vi "Chamber controller Dec 2 2016 new turbo.vi"() -> ()   [LabVIEW 2014]
uses:
  <vilib>/Instr/_visa.llb/VISA Configure Serial Port (Instr).vi
  Environmental Chamber LabVIEW and Instruments/Drivers and Software/Keithley 2100 Series/Public/Configure/Configure 2 Wire Resistance.vi
  <vilib>/Utility/file.llb/Write To Spreadsheet File (string).vi
  <vilib>/Utility/file.llb/Read From Spreadsheet File (string).vi
  Environmental Chamber LabVIEW and Instruments/Drivers and Software/keithley_6430/Keithley 6430/Public/Data/Read (Single Point).vi
  Environmental Chamber LabVIEW and Instruments/Drivers and Software/LabVIEW 8.2 Drivers/keithley_24xx/Keithley 24XX/Public/Data/Read (Single Point).vi
  Environmental Chamber LabVIEW and Instruments/Drivers and Software/keithley_24xx/Keithley 24XX/Keithley 24XX.lvlib
  Environmental Chamber LabVIEW and Instruments/Drivers and Software/keithley_6430/Keithley 6430/Keithley 6430.lvlib
  Environmental Chamber LabVIEW and Instruments/Drivers and Software/Keithley 2100 Series/Keithley 2100 Series.lvlib
panel:
  in  "Arduino COMs":T1={"Arduino 1"="COM23", "Arduino 2"="COM24", "Arduino 3"="COM25", "Arduino 4"="COM26", "Arduino 5"="COM27", "Arduino 6"="COM28"}
  out "saving data?":bool
  out "ArduinoQCM\ncluster":T2 caption="Arduino QCM" {"6" format="%_8g"; "5" format="%_8g"; "4" format="%_8g"; "3" format="%_8g"; "2" format="%_8g"; "1" format="%#_10g"}
  in  "Data logging settings":T3={"Save during sequence only"=TRUE, "Save now"=FALSE, "sec between data points"=0.0, "Current data file path"=path "", "Save sample names"={"QCM1"="", "QCM2"="", "QCM3"="", "QCM4"="", "QCM5"="", "QCM6"="", "SRS"="", "K-2420"="", "K-6430"="", "K-2100"=""}, "Experiment Notes"=""} {"sec between data points" min=0.0 max=30.0 format="%#_13g"}
  in  "Sequence cluster":T4={"Save sequence"=FALSE, "Clear sequence"=FALSE, "Import sequence file"=FALSE, "Tare elapsed time"=TRUE, "Run Sequence"=FALSE, "Stop program when sequence ends"=TRUE, "User-defined\nsequence"=[], "Sequence end time"="", "Sequence\npreview"=[], "Current\nstep"=0} caption="Sequence settings"
  in  "Pressure parameters cluster":T5={"valve % open"=100.0, "Desired pressure"=0.0, "Vapor sccm"=0.0, "Gas sccm"=0.0, "Valve mode"=enum."% Open", "Pressure Mode"=enum."Abs. pressure", "analyte partial pressure"=23.8, "Turbo pump\nauto on"=TRUE, "Valve position (%)"=0.0, "read pressure"=0.0, "read vapor flow"=0.0, "read gas flow"=0.0, "pressure chart"={"pressure"=0.0}} caption="Pressure settings" {"read gas flow" format="%#_3g"; "read vapor flow" format="%#_3g"; "read pressure" format="%#_7f"; "Valve position (%)" format="%#_3g"; "analyte partial pressure" min=0.0 max=100.0 step=5.0; "Gas sccm" min=0 max=200 step=5; "Vapor sccm" min=0 max=200 step=5; "Desired pressure" min=0.0 max=760.0 step=5.0; "valve % open" min=0.0 max=100.0 step=5.0 format="%#_2f"}
  out "J-KEM temp chart":dbl(graph)
  out "Elapsed time (min)":dbl
  out "State date/time":string caption="Start time"
  out "K-2100 (Ohm)":cluster{"Measurement":dbl}(graph) caption="K-2100"
  out "K-6430":cluster{"Measurement":dbl}(graph)
  out "K-2420":cluster{"Resistance":sgl}(graph)
  in  "Gate time (sec)":enum16{"0.1", "1.0 ", "10"}(ring)=enum."1.0 "
  out "Hz":dbl format="%#.7f"
  out "QCM plot":T6(graph)
  in  "Stop":bool
  in  "Clear all charts":bool
  out "O2 sensor output":dbl[](array[numeric]) caption="atm\nTorr"
  in  "rapidox O2 Sensor":bool
  in  "setnag O2 Pump":bool
  in  "Baud Rate 2":i32(ring)=2 items=["2400", "4800", "9600", "19200", "38400", "57600", "115200"]
  in  "Com Port":i32(ring) items=["Com 1", "Com 2", "Com 3", "Com 4", "Com 5", "Com 6", "COM 7", "COM 8", "COM 9", "COM 10", "COM 11", "COM 12", "com 13", "COM 14"]
  in  "Com Port 2":i32(ring) items=["Com 1", "Com 2", "Com 3", "Com 4", "Com 5", "Com 6", "COM 7", "COM 8", "COM 9", "COM 10", "COM 11", "COM 12", "com 13", "COM 14"]
  out "Waveform Chart":cluster{dbl}(graph)
  out "O2 Concentration (PPM)":dbl
  out "Waveform Chart 6":cluster{dbl}(graph)
  # "SRS"
  # "Currently Unused"
  # "100%"
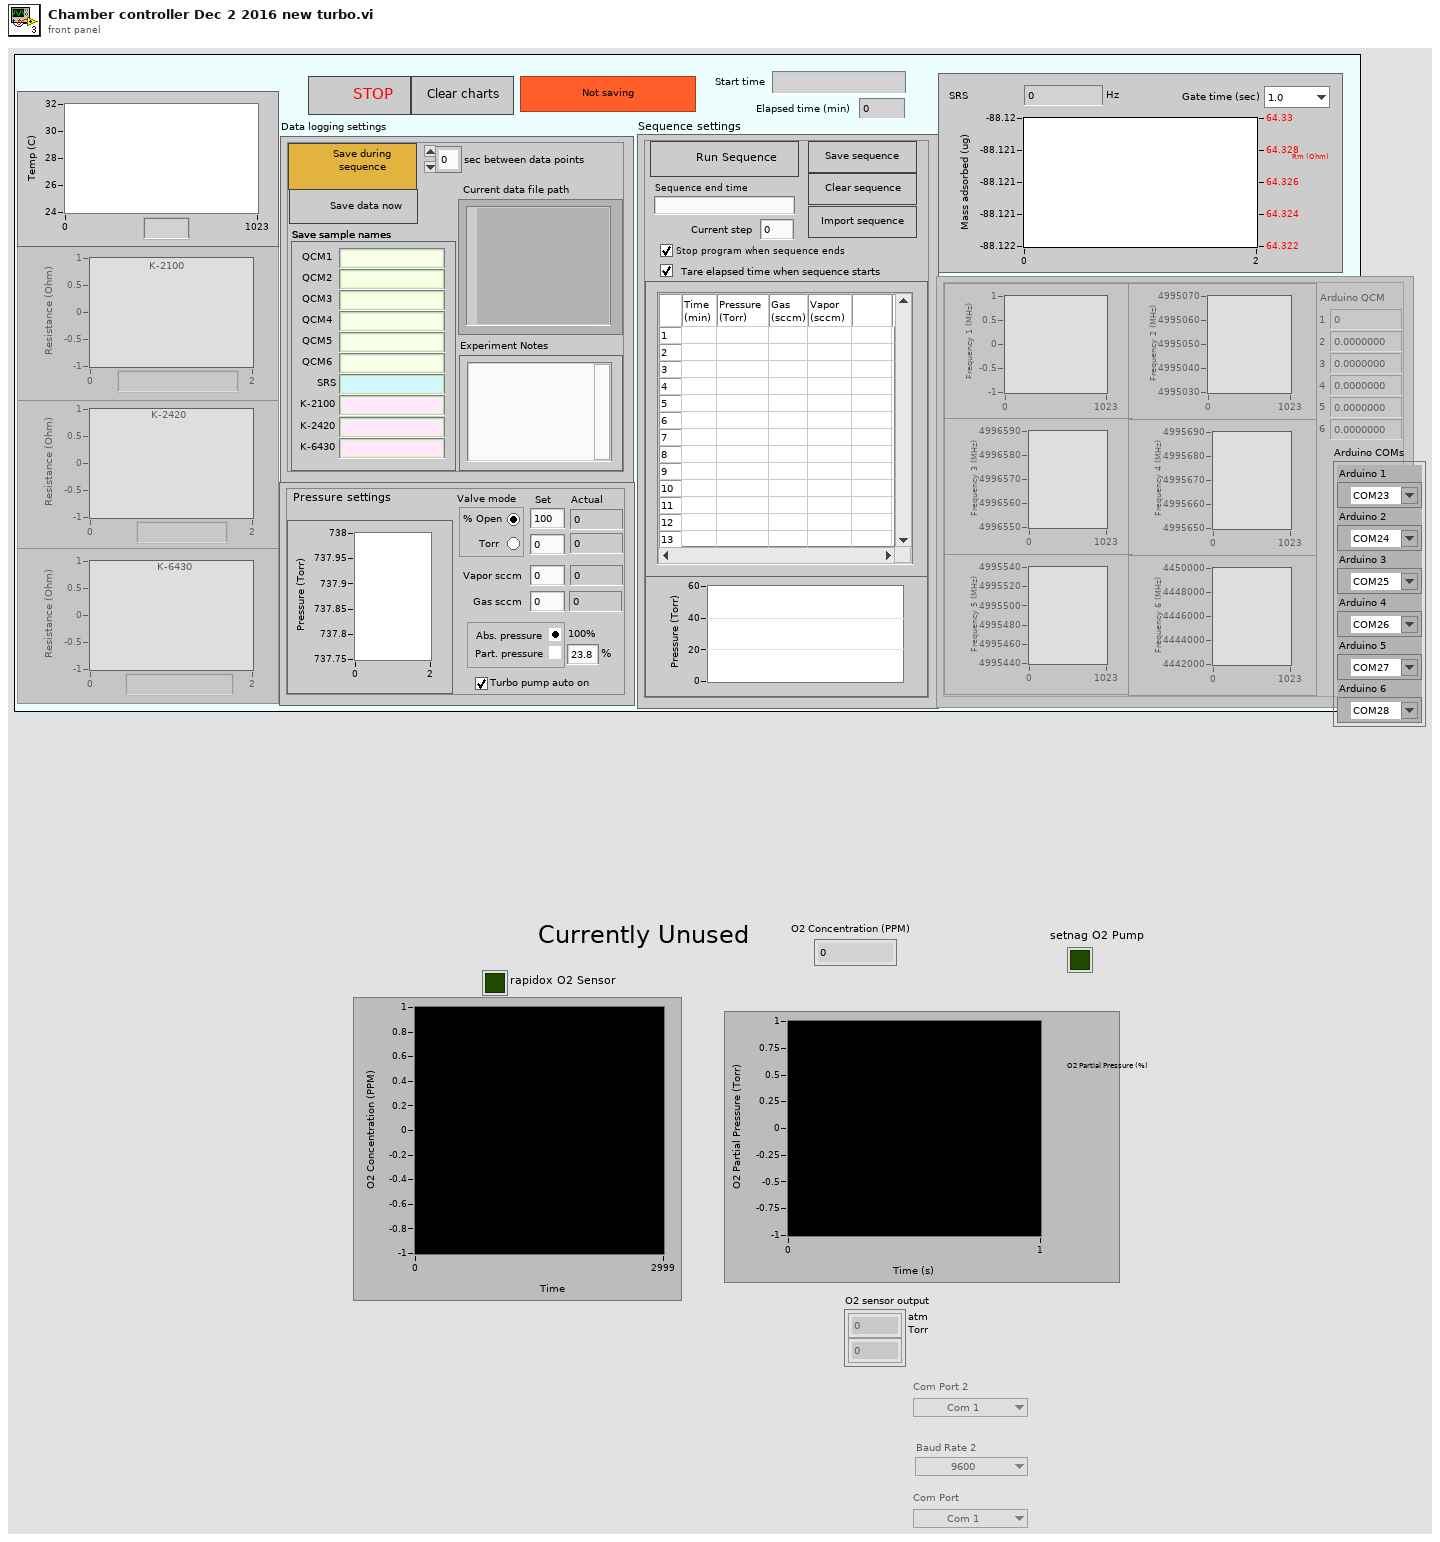
[diagram p1: front panel]
types:
  T1 = cluster{"Arduino 1":refnum<visa-resource-name>, "Arduino 2":refnum<visa-resource-name>, "Arduino 3":refnum<visa-resource-name>, "Arduino 4":refnum<visa-resource-name>, "Arduino 5":refnum<visa-resource-name>, "Arduino 6":refnum<visa-resource-name>}
  T2 = cluster{"arduino qcm 1":dbl, "1":dbl, "arduino qcm 2":dbl, "2":dbl, "arduino qcm 3":dbl, "3":dbl, "arduino qcm 4":dbl, "4":dbl, "arduino qcm 5":dbl, "5":dbl, "arduino qcm 6":dbl, "6":dbl}
  T3 = cluster{"Save during sequence only":bool, "Save now":bool, "sec between data points":dbl, "Current data file path":path, "Save sample names":cluster{"QCM1":string, "QCM2":string, "QCM3":string, "QCM4":string, "QCM5":string, "QCM6":string, "SRS":string, "K-2420":string, "K-6430":string, "K-2100":string}, "Experiment Notes":string}
  T4 = cluster{"Save sequence":bool, "Clear sequence":bool, "Import sequence file":bool, "Tare elapsed time":bool, "Run Sequence":bool, "Stop program when sequence ends":bool, "User-defined\nsequence":string[][], "Sequence end time":string, "Sequence\npreview":cluster{dbl[], dbl[]}[], "Current\nstep":i32}
  T5 = cluster{"valve % open":dbl, "Desired pressure":dbl, "Vapor sccm":sgl, "Gas sccm":sgl, "Valve mode":enum32{"% Open", "Torr "}, "Pressure Mode":enum32{"Abs. pressure", " Part. pressure"}, "analyte partial pressure":dbl, "Turbo pump\nauto on":bool, "Valve position (%)":dbl, "read pressure":dbl, "read vapor flow":dbl, "read gas flow":dbl, "pressure chart":cluster{"pressure":dbl}}
  T6 = cluster{"Numeric Control":dbl, "Resistance out":dbl}
  T7 = cluster{"Keithley 6430":bool, "J-KEM":bool, "Keithley 2420":bool, "Keithley 2100":bool, "SRS QCM":bool, "Pressure control":bool, "Arduino":bool}
  T8 = enum8{"Enabled", "Disabled", "Disabled and Grayed Out"}
  T9 = enum16{"open", "open or create", "create or replace", "create", "open (read only)"}
  T10 = enum16{"no parity", "odd parity", "even parity", "mark parity", "space parity"}
  T11 = cluster{"String":string, "String":string, "String":string}
  T12 = cluster{bool, "task out":refnum<k21>, "error out":errorcluster, "task out":refnum<k21>, "error out":errorcluster, "turbo pump":refnum<visa-resource-name>, "error out":errorcluster}
  T13 = cluster{bool, "task out":refnum<k21>, "error out":errorcluster, "task out":refnum<k21>, "error out":errorcluster, "VISA resource name out":refnum<visa-resource-name>, "error out":errorcluster}
  T14 = cluster{bool, "VISA resource name":refnum<visa-resource-name>, "error out":errorcluster}
  T15 = cluster{bool, "VISA resource name out":refnum<visa-resource-name>, "error out":errorcluster}
  T16 = cluster{"VISA resource name out":refnum<visa-resource-name>, "error out":errorcluster, "VISA resource name out":refnum<visa-resource-name>, "error out":errorcluster, "VISA resource name out":refnum<visa-resource-name>, "error out":errorcluster, "VISA resource name out":refnum<visa-resource-name>, "error out":errorcluster, "VISA resource name out":refnum<visa-resource-name>, "error out":errorcluster, "VISA resource name out 2":refnum<visa-resource-name>, "error out 2":errorcluster}
  T17 = cluster{"Boolean":bool, "VISA resource name out":refnum<visa-resource-name>, "error out":errorcluster}
  T18 = cluster{bool, "VISA out":refnum<visa-resource-name>, "error out":errorcluster}
  T19 = cluster{"Boolean":bool, "VISA out":refnum<visa-resource-name>, "error out":errorcluster}
  T20 = cluster{"Numeric Control":dbl, "Cluster":cluster{"Numeric Control":dbl}, "String":string, "error out":errorcluster}
  T21 = cluster{bool, "Com Port":i32, "Numeric Control out":dbl}
  T22 = cluster{"Arduino address":refnum<visa-resource-name>, "error in (no error)":errorcluster, "Arduino address 2":refnum<visa-resource-name>, "error in (no error) 2":errorcluster, "Arduino address 3":refnum<visa-resource-name>, "error in (no error) 3":errorcluster, "Arduino address 4":refnum<visa-resource-name>, "error in (no error) 4":errorcluster, "Arduino address 5":refnum<visa-resource-name>, "error in (no error) 5":errorcluster, "Arduino address 6":refnum<visa-resource-name>, "error in (no error) 6":errorcluster}
  T23 = cluster{"mean":string, "mean":string, "mean":string, "mean":string, "mean":string, "mean":string}
  T24 = cluster{"String data out":string, string, string, string}
  T25 = cluster{"valve % open":dbl, "Desired pressure":dbl, "Vapor sccm":sgl, "Gas sccm":sgl, "Valve mode":enum32{"% Open", "Torr "}, "Pressure Mode":enum32{"Abs. pressure", " Part. pressure"}, "analyte partial pressure":dbl}
  T26 = cluster{"User-defined\nsequence":string[][], "Present (s)":dbl, "current  step # in":i32, "sequence end time in":timestamp}
  T27 = cluster{"current  step # in":i32, "sequence end time in":timestamp, "Boolean":bool}
  T28 = cluster{"press/RH/gas/vapor":cluster{"pressure":string, "RH":string, "gas flow":string, "vapor flow":string}, "Cluster":cluster{"Valve position (%)":dbl, "read pressure":dbl, "read vapor flow":dbl, "read gas flow":dbl}}
  T29 = cluster{"Boolean":bool, "task out":refnum<k21>, "error out":errorcluster, "task out":refnum<k21>, "error out":errorcluster, "VISA resource name out":refnum<visa-resource-name>, "error out":errorcluster}
  T30 = cluster{"f":dbl, "f":dbl, "f":dbl, "f":dbl, "f":dbl}[]
  T31 = cluster{"pressure":string, "RH":string, "gas flow":string, "vapor flow":string}
  T32 = cluster{"Valve position (%)":dbl, "read pressure":dbl, "read vapor flow":dbl, "read gas flow":dbl}
  T33 = cluster{"mean":dbl, "mean":dbl, "mean":dbl, "mean":dbl, "mean":dbl, "mean":dbl}
  T34 = cluster{"QCM1":string, "QCM2":string, "QCM3":string, "QCM4":string, "QCM5":string, "QCM6":string, "SRS":string, "K-2420":string, "K-6430":string, "K-2100":string}
  T35 = cluster{"mean":dbl, "mean":dbl, "mean":dbl, "mean":dbl, "mean":dbl, "mean":dbl, "mean":dbl, "mean":dbl, "mean":dbl, "mean":dbl, "mean":dbl, "mean":dbl}
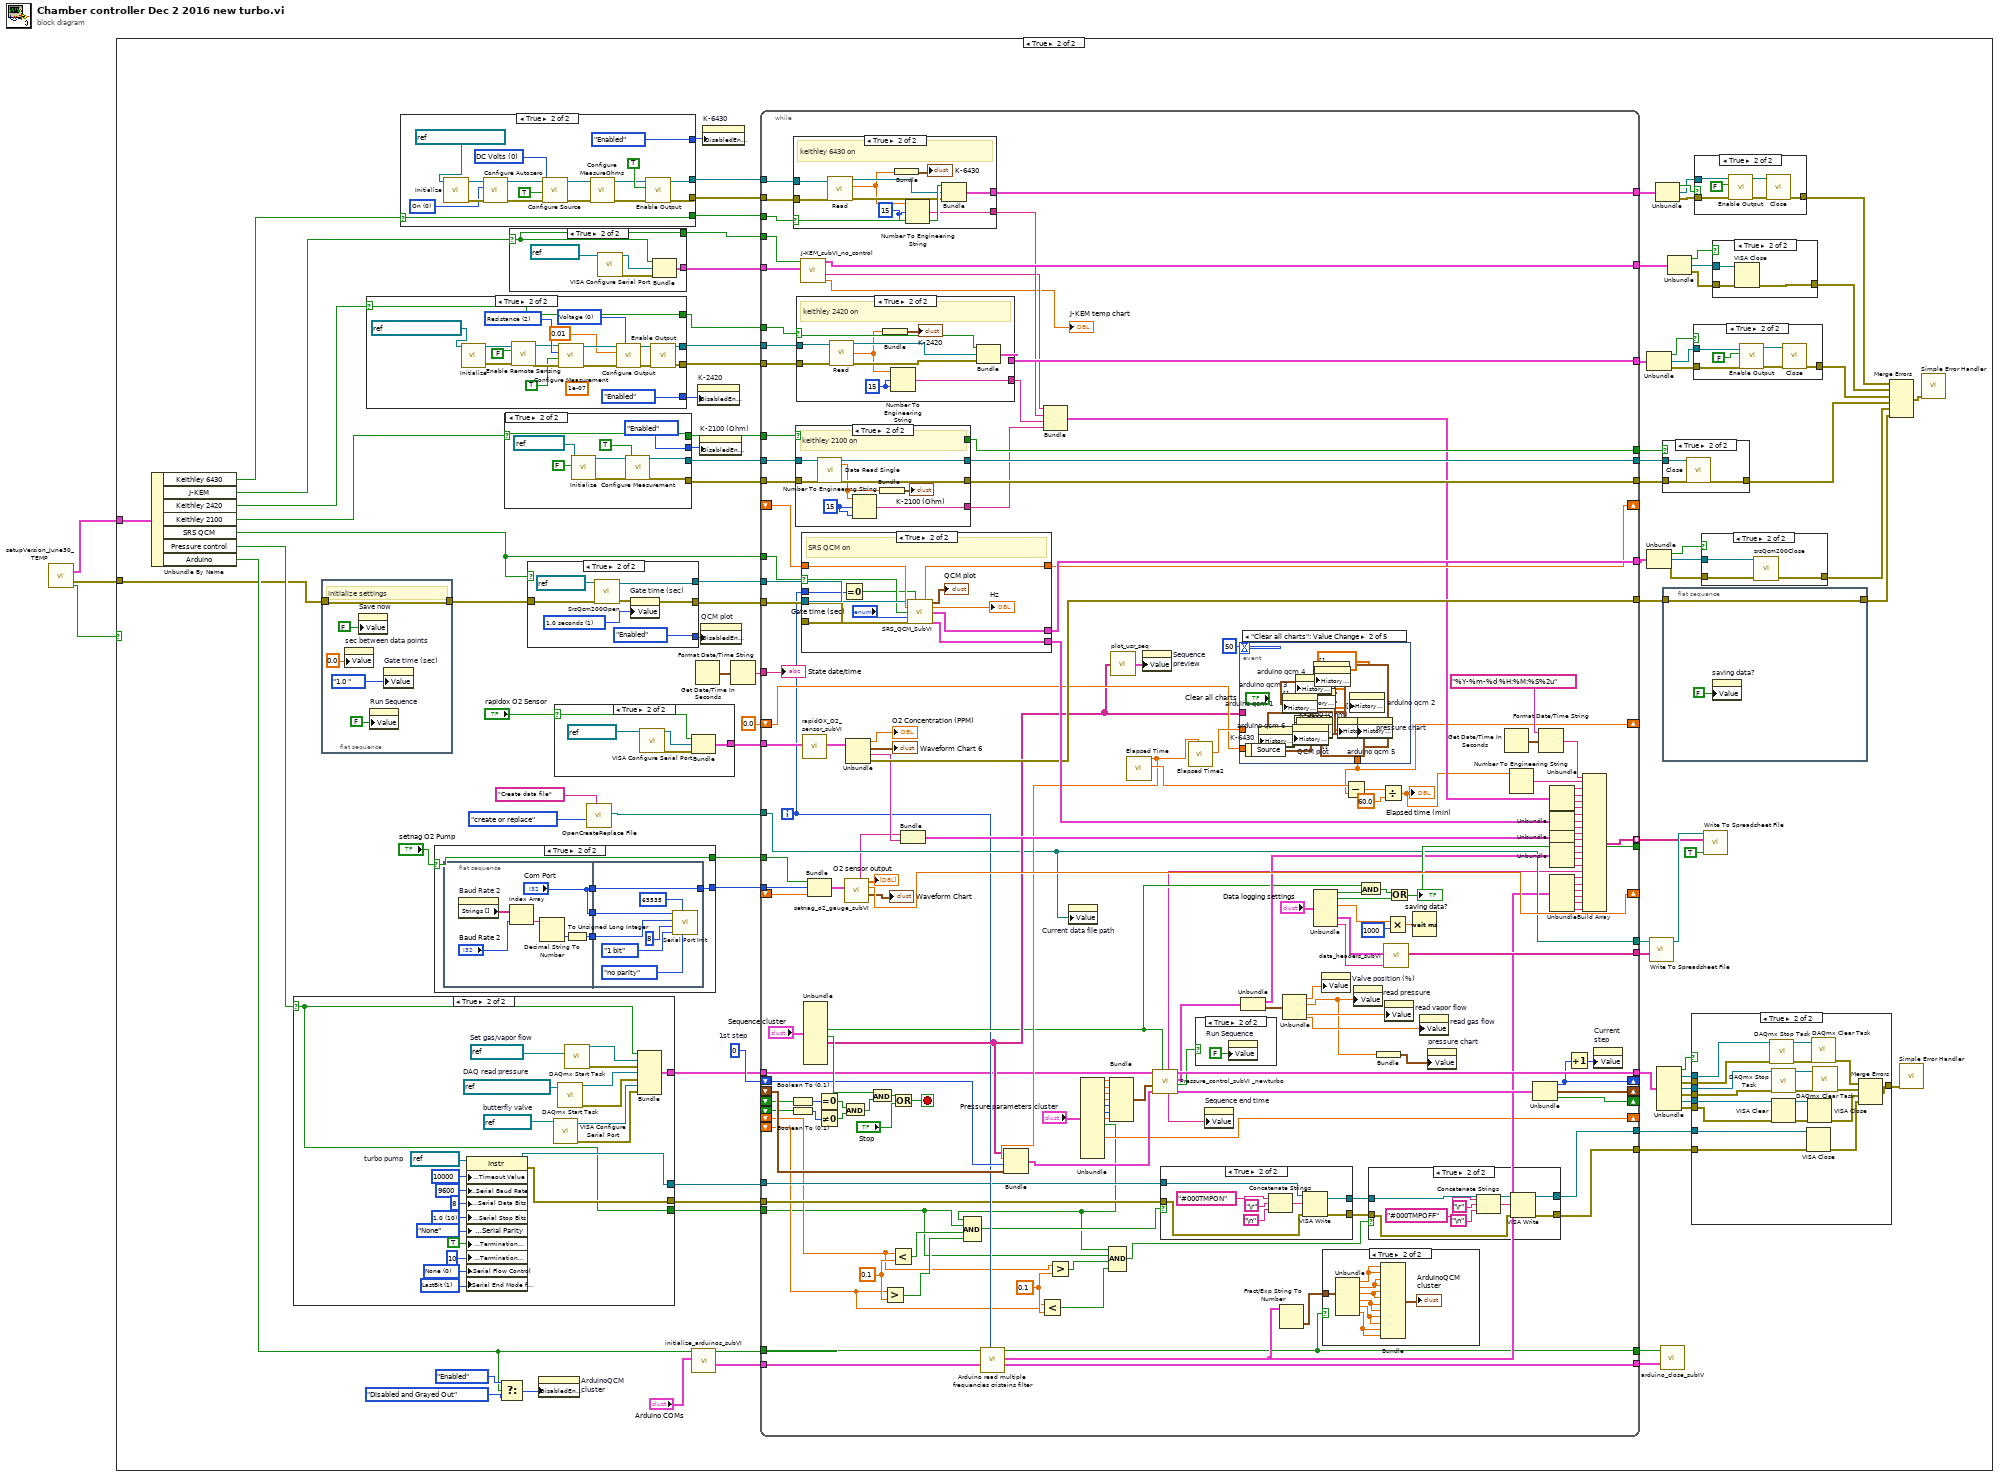
[diagram p0: block diagram]
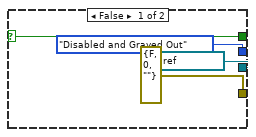
[diagram p4: hidden frame]
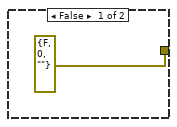
[diagram p5: hidden frame]
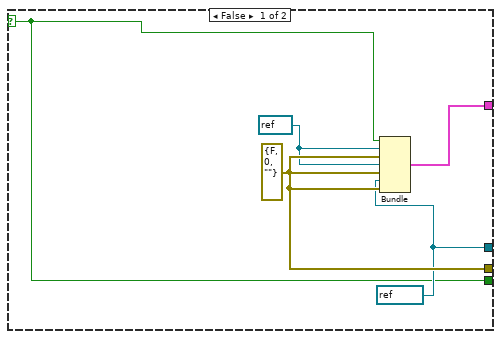
[diagram p6: hidden frame]
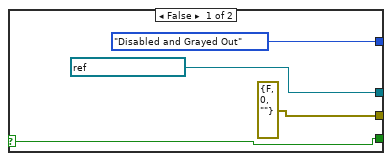
[diagram p8: hidden frame]
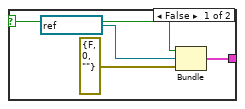
[diagram p9: hidden frame]
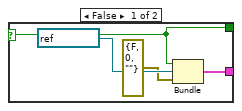
[diagram p11: hidden frame]
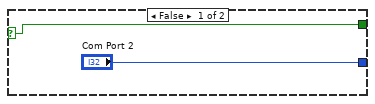
[diagram p12: hidden frame]
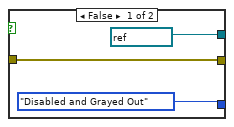
[diagram p14: hidden frame]
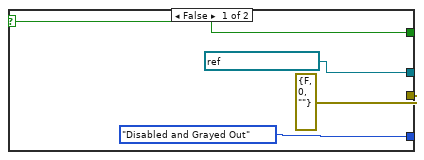
[diagram p16: hidden frame]
diagram:
  n1 = call "setupVersion_June30_TEMP.vi"() -> ("Instruments on/off"=w1:T7, "error IO"=w2:errorcluster, "OK"=w3:bool)  [unwired: 13 in]
  n2 = case shown="True" w3 {
    tunnel: w2 -> [_ w17]
    tunnel: w1 -> [_ w27]
    frame False {
    }
    frame True {
      w34 = 0  # 1st step
      n3 = Unbundle By Name(w27) -> ("Keithley 6430"=w26:bool, "J-KEM"=w25:bool, "Keithley 2420"=w24:bool, "Keithley 2100"=w23:bool, "SRS QCM"=w22:bool, "Pressure control"=w21:bool, "Arduino"=w20:bool)
      n4 = case shown="True" w21 {
        selector: w21 -> [w142 w147]
        tunnel: [w146 w148] -> w15
        tunnel: [w145 w150] -> w7
        tunnel: [w143 w149] -> w8
        tunnel: [w142 w147] -> w6
        frame False {
          w143 = refnum<visa-resource-name> refnum ("turbo pump")
          w144 = refnum<k21> refnum ("task out")
          w145 = errorcluster {"status"=FALSE, "code"=0, "source"=""} ("error out")
          n5 = Bundle(w142, "task out"=w144, "error out"=w145, "task out"=w144, "error out"=w145, "turbo pump"=w143, "error out"=w145) -> (w146:T12)  [unwired: 1 in]
        }
        frame True {
          w154 = u16 1 items=["None", "LastBit", "TermChar"] ("Serial Settings:Serial End Mode for Reads")
          w152 = u16 0 items=["None", "XON/XOFF", "RTS/CTS", "XON/XOFF & RTS/CTS", "DTR/DSR", "XON/XOFF & DTR/DSR"] ("flow control (0:none)")
          w155 = u16 10 items=["1.0"=10, "1.5"=15, "2.0"=20] ("stop bits (10: 1 bit)")
          w151 = refnum<visa-resource-name> "COM7"  # turbo pump
          w167 = refnum<visa-resource-name> "COM5"  # butterfly valve
          w168 = refnum<k21> "Setflow"  # Set gas/vapor flow
          w169 = refnum<k21> "AllDaqReadings"  # DAQ read pressure
          n6 = property class="Instr"(reference=w151, "General Settings:Timeout Value"=u32 10000 ("timeout (10sec)"), "Serial Settings:Serial Baud Rate"=u32 9600 ("baud rate (9600)"), "Serial Settings:Serial Data Bits"=u16 8 ("data bits (8)"), "Serial Settings:Serial Stop Bits"=w155, "Serial Settings:Serial Parity"=enum16{"None", "Odd", "Even", "Mark", "Space"}."None" ("parity (0:none)"), "Message Based Settings:Termination Character Enable"=TRUE ("Enable Termination\nChar (T)"), "Message Based Settings:Termination Character"=u8 10 ("termination char\n(0xA = '\\n' = LF)"), "Serial Settings:Serial Flow Control"=w152, "Serial Settings:Serial End Mode for Reads"=w154) -> (reference out=w149:refnum<visa-resource-name>, error out=w150:errorcluster)  [unwired: 1 in]
          n7 = call-poly "VISA Configure Serial Port"("VISA resource name"=w167) -> ("VISA resource name out"=w162:refnum<visa-resource-name>, "error out"=w161:errorcluster)  [unwired: 13 in]
          n8 = call <vilib>:"DAQmx Start Task.vi"("task/channels in"=w169) -> ("task out"=w164:refnum<k21>, "error out"=w163:errorcluster)  [unwired: 13 in]
          n9 = call <vilib>:"DAQmx Start Task.vi"("task/channels in"=w168) -> ("task out"=w166:refnum<k21>, "error out"=w165:errorcluster)  [unwired: 13 in]
          n10 = Bundle(w147, "task out"=w166, "error out"=w165, "task out"=w164, "error out"=w163, "VISA resource name out"=w162, "error out"=w161) -> (w148:T13)  [unwired: 1 in]
        }
      }
      n11 = flat-sequence {
        tunnel: [w98] -> w16
        tunnel: w17 -> [w98]
        frame #0 {
          # "initialize settings"
          n12 = property on="sec between data points" class="DigNum (strict)"("Value"=0.0) -> ()  [unwired: 2 in, 2 out]
          n13 = property on="Save now" class="Bool (strict)"("Value"=FALSE) -> ()  [unwired: 2 in, 2 out]
          n14 = property on="Run Sequence" class="Bool (strict)"("Value"=FALSE) -> ()  [unwired: 2 in, 2 out]
          n15 = property on="Gate time (sec)" class="Enum (strict)"("Value"=enum16{"0.1", "1.0 ", "10"}."1.0 " ("Gate time (sec)")) -> ()  [unwired: 2 in, 2 out]
        }
      }
      n16 = case shown="True" w24 {
        selector: w24 -> [w261 w265]
        tunnel: [refnum<visa-resource-name> "GPIB1::24::INSTR" ("VISA resource name") w274] -> w95
        tunnel: [errorcluster {"status"=FALSE, "code"=0, "source"=""} ("error out") w269] -> w94
        tunnel: [T8."Disabled and Grayed Out" ("Disabled") T8."Enabled" ("Disabled")] -> w58
        tunnel: [w261 w265] -> w51
        frame False {
        }
        frame True {
          (unwired) 1e-07 ("Manual Range (1.0)")
          w276 = u16 0 items=["Voltage", "Current"] ("Source Mode  (0: Voltage)")
          w281 = u16 2 items=["Volts", "Current", "Resistance"] ("Function (0: Volts)")
          n17 = call "Initialize.vi"("VISA resource name"=refnum<visa-resource-name> "GPIB1::24::INSTR") -> ("error out"=w270:errorcluster, "VISA resource name out"=w273:refnum<visa-resource-name>)  [unwired: 9 in]
          n18 = call "Enable Remote Sensing.vi"("error in (no error)"=w270, "Enable Remote Sensing (T: Enable)"=FALSE ("4-wire?"), "VISA resource name"=w273) -> ("error out"=w271:errorcluster, "VISA resource name out"=w272:refnum<visa-resource-name>)  [unwired: 7 in]
          n19 = call "Configure Measurement.vi"("error in (no error)"=w271, "Enable Auto Range (T:Enable)"=TRUE, "Function (0: Volts)"=w281, "VISA resource name"=w272) -> ("error out"=w280:errorcluster, "VISA resource name out"=w279:refnum<visa-resource-name>)  [unwired: 6 in]
          n20 = call "Configure Output.vi"("Source Mode  (0: Voltage)"=w276, "error in (no error)"=w280, "Output Level (0)"=0.01 ("Applied Voltage (V)"), "VISA resource name"=w279) -> ("error out"=w278:errorcluster, "VISA resource name out"=w277:refnum<visa-resource-name>)  [unwired: 6 in]
          n21 = call "Enable Output.vi"("error in (no error)"=w278, "VISA resource name"=w277) -> ("error out"=w269:errorcluster, "VISA resource name out"=w274:refnum<visa-resource-name>)  [unwired: 8 in]
        }
      }
      n22 = case shown="True" w26 {
        selector: w26 -> [w177 w181]
        tunnel: [refnum<visa-resource-name> "GPIB0::29::INSTR" ("VISA resource name") w192] -> w64
        tunnel: [errorcluster {"status"=FALSE, "code"=0, "source"=""} ("error out") w193] -> w63
        tunnel: [T8."Disabled and Grayed Out" ("Disabled") T8."Enabled" ("Disabled")] -> w57
        tunnel: [w177 w181] -> w50
        frame False {
        }
        frame True {
          w182 = u16 0 items=["DC Volts", "DC Current"] ("Source Function (0: DC Volts)")
          w189 = u16 0 items=["On", "Off", "Once"] ("Autozero  (0: On)")
          n23 = call "Initialize.vi"("VISA resource name"=refnum<visa-resource-name> "GPIB0::29::INSTR") -> ("error out"=w190:errorcluster, "VISA resource name out"=w191:refnum<visa-resource-name>)  [unwired: 4 in, 5 out]
          n24 = call "Configure Autozero.vi"("error in (no error)"=w190, "Autozero  (0: On)"=w189, "VISA resource name"=w191) -> ("error out"=w185:errorcluster, "VISA resource name out"=w187:refnum<visa-resource-name>)  [unwired: 7 in]
          n25 = call "Configure Source.vi"("error in (no error)"=w185, "Auto Range (T:Enable)"=TRUE, "Source Function (0: DC Volts)"=w182, "VISA resource name"=w187) -> ("error out"=w184:errorcluster, "VISA resource name out"=w186:refnum<visa-resource-name>)  [unwired: 6 in]
          n26 = call "Configure MeasureOhms.vi"("error in (no error)"=w184, "VISA resource name"=w186) -> ("error out"=w197:errorcluster, "VISA resource name out"=w195:refnum<visa-resource-name>)  [unwired: 4 in, 4 out]
          n27 = call "Enable Output.vi"("error in (no error)"=w197, "Enable Output (F:Off)"=TRUE ("Output (F:Off)"), "VISA resource name"=w195) -> ("error out"=w193:errorcluster, "VISA resource name out"=w192:refnum<visa-resource-name>)  [unwired: 7 out]
        }
      }
      n28 = case shown="True" "setnag O2 Pump" {
        selector: "setnag O2 Pump" -> [w220 w222]
        tunnel: ["Com Port 2" w223] -> w91
        tunnel: [w220 w222] -> w39
        frame False {
        }
        frame True {
          n29 = flat-sequence {
            tunnel: ["Com Port"] -> w226
            tunnel: [w228] -> w225
            tunnel: ["Com Port"] -> w224
            tunnel: w226 -> [w234]
            tunnel: w225 -> [w233]
            tunnel: w224 -> [w235]
            tunnel: [w235] -> w223
            frame #0 {
              n30 = property on="Baud Rate 2" class="Ring (strict)"() -> ("Strings []"=w230:string[])  [unwired: 2 in, 2 out]
              n31 = Index Array(array=w230, index="Baud Rate 2") -> (element=w231:string)
              n32 = Decimal String To Number(string=w231) -> (number=w229:i32)  [unwired: 2 in, 1 out]
              n33 = To Unsigned Long Integer(number=w229) -> (unsigned 32bit integer=w228:u32)
            }
            frame #1 {
              n34 = call <vilib>:"Serial Port Init.vi"("parity"=T10."no parity", "buffer size"=u16 65535, "stop bits"=enum16{"1 bit", "1.5 bits", "2 bits"}."1 bit", "data bits"=u16 8, "baud rate"=w233, "port number"=w234) -> ()  [unwired: 1 in, 1 out]
            }
          }
        }
      }
      n35 = Select(t=T8."Enabled" ("Disabled"), s=w20, f=T8."Disabled and Grayed Out" ("Disabled")) -> (s? t:f=w31:T8)
      n36 = case shown="True" w23 {
        selector: w23 -> [w110 w115]
        tunnel: [refnum<visa-resource-name> "K-2100" ("VISA resource name out") w118] -> w48
        tunnel: [errorcluster {"status"=FALSE, "code"=0, "source"=""} ("error out") w117] -> w47
        tunnel: [w110 w115] -> w46
        tunnel: [T8."Disabled and Grayed Out" ("Disabled") T8."Enabled" ("Disabled")] -> w41
        frame False {
        }
        frame True {
          n37 = call "Initialize.vi"("VISA resource name"=refnum<visa-resource-name> "K-2100", "Reset? (T: Reset)"=FALSE) -> ("VISA resource name out"=w119:refnum<visa-resource-name>, "error out"=w116:errorcluster)  [unwired: 16 in]
          n38 = call-poly "Configure Measurement.vi"("VISA resource name"=w119, "error in (no error)"=w116, "Auto Range? (T: Auto)"=TRUE) -> ("VISA resource name out"=w118:refnum<visa-resource-name>, "error out"=w117:errorcluster)  [unwired: 15 in]
        }
      }
      n39 = case shown="True" w25 {
        selector: w25 -> [w211 w216]
        tunnel: [w212 w217] -> w80
        tunnel: [w211 w216] -> w74
        frame False {
          n40 = Bundle(w211, "VISA resource name"=refnum<visa-resource-name> "COM3", "error out"=errorcluster {"status"=FALSE, "code"=0, "source"=""}) -> (w212:T14)  [unwired: 1 in]
        }
        frame True {
          n41 = call-poly "VISA Configure Serial Port"("VISA resource name"=refnum<visa-resource-name> "COM3") -> ("VISA resource name out"=w218:refnum<visa-resource-name>, "error out"=w215:errorcluster)  [unwired: 13 in]
          n42 = Bundle(w216, "VISA resource name out"=w218, "error out"=w215) -> (w217:T15)  [unwired: 1 in]
        }
      }
      n43 = case shown="True" w22 {
        tunnel: [refnum<visa-resource-name> "COM6" ("VISA in") w250] -> w93
        tunnel: [w245 w247] -> w92
        tunnel: w16 -> [w245 w252]
        tunnel: [T8."Disabled and Grayed Out" ("Disabled") T8."Enabled" ("Disabled")] -> w59
        frame False {
        }
        frame True {
          w249 = u16 1 items=["0.1 seconds", "1.0 seconds", "10.0 seconds"] ("Gate time")
          n44 = call "SrsQcm200Open.vi"("error in"=w252, "VISA in"=refnum<visa-resource-name> "COM6") -> ("error out"=w248:errorcluster, "VISA out"=w250:refnum<visa-resource-name>)  [unwired: 3 in]
          n45 = property on="Gate time (sec)" class="Enum (strict)"(error in=w248, "Value"=w249) -> (error out=w247:errorcluster)  [unwired: 1 in, 1 out]
        }
      }
      n46 = property on="ArduinoQCM\ncluster" class="Clust (strict)"("DisabledEnum"=w31) -> ()  [unwired: 2 in, 2 out]
      n47 = case shown="True" "rapidox O2 Sensor" {
        selector: "rapidox O2 Sensor" -> [w198 w203]
        tunnel: [w199 w204] -> w70
        frame False {
          n48 = Bundle(w198, "VISA resource name"=refnum<visa-resource-name> "COM7", "error out"=errorcluster {"status"=FALSE, "code"=0, "source"=""}) -> (w199:T14)  [unwired: 1 in]
        }
        frame True {
          n49 = call-poly "VISA Configure Serial Port"("VISA resource name"=refnum<visa-resource-name> "COM7") -> ("VISA resource name out"=w205:refnum<visa-resource-name>, "error out"=w202:errorcluster)  [unwired: 13 in]
          n50 = Bundle(w203, "VISA resource name out"=w205, "error out"=w202) -> (w204:T15)  [unwired: 1 in]
        }
      }
      n51 = call "OpenCreateReplace File.vi"("prompt"="Create data file", "function (open:0)"=T9."create or replace") -> ("new file path"=w49:path)  [unwired: 6 in, 3 out]
      n52 = call "initialize_arduinos_subVI.vi"("arduino 1-6 addresses"="Arduino COMs", "arduinos on?"=w20) -> ("arduino addresses/errors"=w35:T16, "arduinos on/off"=w55:bool)  [unwired: 8 in]
      n53 = Get Date/Time In Seconds() -> (seconds since 1Jan1904=w97:timestamp)
      n54 = property on="K-2420" class="WFChart (strict)"("DisabledEnum"=w58) -> ()  [unwired: 2 in, 2 out]
      n55 = property on="K-2100 (Ohm)" class="WFChart (strict)"("DisabledEnum"=w41) -> ()  [unwired: 2 in, 2 out]
      n56 = property on="QCM plot" class="WFChart (strict)"("DisabledEnum"=w59) -> ()  [unwired: 2 in, 2 out]
      n57 = property on="K-6430" class="WFChart (strict)"("DisabledEnum"=w57) -> ()  [unwired: 2 in, 2 out]
      n58 = Format Date/Time String(seconds (now)=w97) -> (date/time string=w38:string)  [unwired: 2 in]
      n59 = while {
        shift-right: [w443] -> _
        shift-left: _ -> [w374]
        tunnel: [w427] -> w56 mode=indexing if=w396
        tunnel: w51 -> [w432]
        tunnel: w95 -> [w442]
        tunnel: w94 -> [w441]
        tunnel: w93 -> [w440]
        tunnel: w92 -> [w439]
        tunnel: w22 -> [w438]
        tunnel: w39 -> [w376]
        tunnel: w91 -> [w377]
        tunnel: [w437] -> w88
        tunnel: [w436] -> w84
        tunnel: w80 -> [w435]
        tunnel: [w434] -> w79
        tunnel: w74 -> [w433]
        tunnel: w70 -> [w385]
        tunnel: [w381] -> w19
        tunnel: [w318] -> w69
        tunnel: w49 -> [w318]
        shift-right: [w425] -> _
        shift-left: _ -> [w426]
        tunnel: w64 -> [w431]
        tunnel: w63 -> [w430]
        tunnel: [w429] -> w62
        tunnel: [w396] -> _
        tunnel: w55 -> [w306]
        tunnel: w35 -> [w309]
        tunnel: [w305] -> w53
        tunnel: [w307] -> w54
        tunnel: [w413] -> w52
        tunnel: w50 -> [w408]
        tunnel: w48 -> [w395]
        tunnel: w47 -> [w394]
        tunnel: w46 -> [w393]
        tunnel: [w392] -> w45
        tunnel: [w391] -> w44
        tunnel: [w390] -> w43
        shift-right: [w368] -> _
        shift-left: 0.0 ("Elapsed Time (s)") -> [w369]
        tunnel: w38 -> [w359]
        tunnel: w15 -> [w302]
        shift-right: [w314] -> _
        shift-left: w34 -> [w332]
        shift-right: [w338] -> _
        shift-left: _ -> [w336]
        shift-right: [w337] -> _
        shift-left: _ -> [w335]
        shift-left: _ -> [w334]
        tunnel: [w330] -> w33
        tunnel: w8 -> [w297]
        tunnel: w7 -> [w296]
        tunnel: w6 -> [w286]
        tunnel: [w291] -> w5
        tunnel: [w292] -> w4
        shift-right: [w301] -> _
        shift-left: _ -> [w288]
        shift-left: _ -> [w287]
        i -> [w304]
        stop <- w398 stop-if-true
        w290 = 0.1 ("y")
        w300 = 0.1 ("y")
        n60 = Boolean To (0,1)(Boolean=w335) -> (0, 1=w406:i16)
        n61 = Boolean To (0,1)(Boolean=w334) -> (0, 1=w405:i16)
        n62 = case "Keithley 6430" shown="True" w408 {
          selector: w408 -> [w498 w509]
          tunnel: w431 -> [w497 w506]
          tunnel: w430 -> [w496 w505]
          tunnel: ["" w508] -> w380
          tunnel: [w495 w507] -> w429
          frame False {
            # "keithley 6430 off"
            n63 = Bundle(w498, "VISA resource name out"=w497, "error out"=w496) -> (w495:T15)  [unwired: 1 in]
          }
          frame True {
            w500 = i16 15 ("width (-)")
            # "keithley 6430 on"
            n64 = call-poly "Read.vi"("error in (no error)"=w505, "VISA resource name"=w506) -> ("error out"=w504:errorcluster, "Measurement"=w502:dbl, "VISA resource name out"=w503:refnum<visa-resource-name>)  [unwired: 1 in, 6 out]
            n65 = Bundle("Measurement"=w502) -> (→"K-6430":cluster{"Measurement":dbl})  [unwired: 1 in]
            n66 = Number To Engineering String(2:w500, 3:w500, 4:w502) -> (0:w508:string)  [unwired: 1 in]
            n67 = Bundle(w509, "VISA resource name out"=w503, "error out"=w504) -> (w507:T15)  [unwired: 1 in]
          }
        }
        n68 = case shown="True" w393 {
          selector: w393 -> [w474 w479]
          tunnel: [w475 w486] -> w391
          tunnel: [w476 w485] -> w390
          tunnel: w395 -> [w475 w484]
          tunnel: w394 -> [w476 w483]
          tunnel: ["" w481] -> w378
          tunnel: [w474 w479] -> w392
          frame False {
            # "keithley 2100 off"
          }
          frame True {
            w478 = i16 15 ("width (-)")
            # "keithley 2100 on"
            n69 = call "Data Read Single.vi"("VISA resource name"=w484, "error in (no error)"=w483) -> ("VISA resource name out"=w486:refnum<visa-resource-name>, "Measurement"=w482:dbl, "error out"=w485:errorcluster)  [unwired: 15 in]
            n70 = Number To Engineering String ("elapsed time (min)")(2:w478, 3:w478, 4:w482) -> (0:w481:string)  [unwired: 1 in]
            n71 = Bundle("Measurement"=w482) -> (→"K-2100 (Ohm)":cluster{"Measurement":dbl})  [unwired: 1 in]
          }
        }
        n72 = case "Keithley 2420" shown="True" w432 {
          selector: w432 -> [w513 w522]
          tunnel: w442 -> [w512 w517]
          tunnel: w441 -> [w511 w516]
          tunnel: [w510 w520] -> w437
          tunnel: ["" w519] -> w379
          frame False {
            # "keithley 2420 off"
            n73 = Bundle(w513, "VISA resource name out"=w512, "error out"=w511) -> (w510:T15)  [unwired: 1 in]
          }
          frame True {
            w515 = i16 15 ("width (-)")
            # "keithley 2420 on"
            n74 = call-poly "Read.vi"("VISA resource name"=w517, "error in (no error)"=w516) -> ("VISA resource name out"=w523:refnum<visa-resource-name>, "Resistance"=w518:sgl, "error out"=w521:errorcluster)  [unwired: 7 in, 4 out]
            n75 = Bundle("Resistance"=w518) -> (→"K-2420":cluster{"Resistance":sgl})  [unwired: 1 in]
            n76 = Number To Engineering String(2:w515, 3:w515, 4:w518) -> (0:w519:string)  [unwired: 1 in]
            n77 = Bundle(w522, "VISA resource name out"=w523, "error out"=w521) -> (w520:T15)  [unwired: 1 in]
          }
        }
        n78 = call "J-KEM_subVI_no_control.vi"("Address in"=w435, "J-KEM on?"=w433) -> ("Temp (C)"=→"J-KEM temp chart":dbl, "String data out"=w367:string, "Address out"=w434:T17)  [unwired: 6 in, 1 out]
        n79 = case "SRS QCM" shown="True" w438 {
          selector: w438 -> [w527 w536]
          tunnel: w440 -> [w530 w538]
          tunnel: w439 -> [w529 w539]
          tunnel: [w528 w542] -> w436
          tunnel: w426 -> [w525 w541]
          tunnel: [w525 w540] -> w425
          tunnel: [T11 {"String"="", "String"="", "String"=""} ("M,F,MR output cluster") w535] -> w418
          tunnel: w304 -> [_ w532]
          frame False {
            # "SRS QCM off"
            n80 = Bundle(w527, "VISA out"=w530, "error out"=w529) -> (w528:T18)  [unwired: 1 in]
          }
          frame True {
            # "SRS QCM on"
            n81 = Equal To 0?(x=w532) -> (x = 0?=w533:bool)
            n82 = call "SRS_QCM_SubVI.vi"("VISA Refnum in"=w538, "first iteration?"=w533, "Frequency out 3"=w541, "Boolean 2"=w536, "Gate time"="Gate time (sec)", "error in (no error)"=w539) -> ("Frequency out 2"=w540:dbl, "Cluster"=→"QCM plot":T6, "Frequency out"=→"Hz":dbl, "Cluster 2"=w542:T19, "M,F,MR output cluster"=w535:T11)  [unwired: 2 in, 3 out]
          }
        }
        n83 = call "rapidOX_O2_sensor_subVI.vi"("rapid ox info in"=w385) -> ("rapidox info out"=w384:T20)  [unwired: 10 in]
        n84 = Unbundle("Sequence cluster") -> ("Run Sequence"=w324:bool, "Stop program when sequence ends"=w333:bool, "User-defined\nsequence"=w328:string[][])  [unwired: 7 out]
        n85 = Bundle(w376, "Com Port"=w377, "Numeric Control out"=w374) -> (w375:T21)  [unwired: 1 in]
        n86 = Equal To 0?(x=w406) -> (x = 0?=w403:bool)
        n87 = Not Equal To 0?(x=w405) -> (x != 0?=w404:bool)
        n88 = And(x=w403, y=w404) -> (x .and. y?=w397:bool)
        n89 = call "setnag_o2_gauge_subVI.vi"("setnag info in"=w375) -> ("Cluster"=→"Waveform Chart":cluster{"Numeric Control":dbl}, "Numeric Control out"=w443:dbl, "Array"=→"O2 sensor output":dbl[], "String"=w315:string)  [unwired: 7 in]
        n90 = Unbundle(w384) -> ("Numeric Control"=→"O2 Concentration (PPM)":dbl, "Cluster"=→"Waveform Chart 6":cluster{"Numeric Control":dbl}, "String"=w358:string, "error out"=w381:errorcluster)
        n91 = And(x=w333, y=w397) -> (x .and. y?=w372:bool)
        n92 = Greater?(x=w287, y=w300) -> (0:w299:bool)
        n93 = Less?(x=w288, y=w300) -> (x < y?=w298:bool)
        n94 = Or(x=w372, y="Stop") -> (x .or. y?=w398:bool)
        n95 = Bundle("String"=w315, "String"=w358) -> (w357:cluster{"String":string, "String":string})  [unwired: 1 in]
        n96 = call "Arduino read multiple frequencies cristains filter.vi"("main loop iteration number"=w304, "arduino addresses in"=w309, "arduinos on?"=w306) -> ("arduino addresses out"=w307:T22, "arduino frequencies out"=w308:T23, "arduinos on"=w305:bool)  [unwired: 6 in]
        n97 = Less?(x=w287, y=w290) -> (x < y?=w284:bool)
        n98 = Bundle("String data out"=w367, w380, w379, w378) -> (w373:T24)  [unwired: 1 in]
        n99 = Greater?(x=w288, y=w290) -> (0:w285:bool)
        n100 = property on="Current data file path" class="Path"("Value"=w318) -> ()  [unwired: 2 in, 2 out]
        n101 = Unbundle("Pressure parameters cluster") -> ("valve % open"=w347:dbl, "Desired pressure"=w349:dbl, "Vapor sccm"=w350:sgl, "Gas sccm"=w351:sgl, "Valve mode"=w352:enum32{"% Open", "Torr "}, "Pressure Mode"=w353:enum32{"Abs. pressure", " Part. pressure"}, "analyte partial pressure"=w354:dbl, "Turbo pump\nauto on"=w289:bool, "read pressure"=w301:dbl)  [unwired: 4 out]
        n102 = Compound Arithmetic op=AND(w289, w286, w298, w299) -> (w295:bool)
        n103 = Compound Arithmetic op=AND(w289, w286, w285, w284) -> (w283:bool)
        n104 = Bundle("valve % open"=w347, "Desired pressure"=w349, "Vapor sccm"=w350, "Gas sccm"=w351, "Valve mode"=w352, "Pressure Mode"=w353, "analyte partial pressure"=w354) -> (w346:T25)  [unwired: 1 in]
        n105 = call "plot_usr_seq.vi"("User-defined sequence"=w328) -> ("Sequence Preview"=w320:cluster{dbl[], dbl[]}[])
        n106 = call "Elapsed Time"() -> ("Present (s)"=w340:dbl, "Elapsed Time (s)"=w387:dbl)  [unwired: 12 in, 6 out]
        n107 = Bundle("User-defined\nsequence"=w328, "Present (s)"=w340, "current  step # in"=w332, "sequence end time in"=w336) -> (w341:T26)  [unwired: 1 in]
        n108 = property on="Sequence\npreview" class="XYGraph (strict)"("Value"=w320) -> ()  [unwired: 2 in, 2 out]
        n109 = call "Pressure_control_subVI _newturbo.vi"("Run Sequence"=w324, "user sequence, present (s) in, current step in, seq time in"=w341, "pressure parameters in"=w346, "pressure control on?/daq IDs/errors"=w302) -> ("current step # out, shift register time out, seq button on?"=w339:T27, "sequence over? USE THIS TO REINITIALIZE RUN SEQUENCE BUTTON SO PROGRAM ENDS"=w329:bool, "save press/RH/gasflow/vaporflow - read valve position/pressure/vaporflow/gasflow"=w327:T28, "pressure control on?/daq IDs/errors out"=w330:T29, "sequence end date/time string"=w331:string, "pressure_setpoint"=w311:string)  [unwired: 2 in]
        n110 = case shown="True" w295 {
          tunnel: w297 -> [w456 w459]
          tunnel: w296 -> [w455 w460]
          tunnel: [w456 w458] -> w294
          tunnel: [w455 w457] -> w293
          frame False {
          }
          frame True {
            n111 = Concatenate Strings("#000TMPON" ("write buffer 2"), "\r", "\n") -> (w461:string)
            n112 = VISA Write(VISA resource name=w459, write buffer=w461, error in (no error)=w460) -> (VISA resource name out=w458:refnum<visa-resource-name>, error out=w457:errorcluster)  [unwired: 1 out]
          }
        }
        n113 = call "Elapsed Time2"("Set Start Time (s)"=w340) -> ("Elapsed Time (s)"=w370:dbl)  [unwired: 11 in, 7 out]
        n114 = case shown="True" w329 {
          frame False {
          }
          frame True {
            n115 = property on="Run Sequence" class="Bool (strict)"("Value"=FALSE ("Run Sequence")) -> ()  [unwired: 2 in, 2 out]
          }
        }
        n116 = property on="Sequence end time" class="Str"("Value"=w331) -> ()  [unwired: 2 in, 2 out]
        n117 = event shown="[1] \"Clear all charts\": Value Change" {
          selector: _ -> [_ _ _ _ _]
          dyn-events: _ -> [_ _ _ _ _]
          timeout: 50 -> [_ _ _ _ _]
          tunnel: w328 -> [_ _ _ w493 _]
          tunnel: w370 -> [_ _ _ _ _]
          tunnel: w369 -> [w487 _ _ _ _]
          tunnel: [w487 _ _ _ _] -> w368
          event Timeout {
            n118 = event-data() -> ()  [unwired: 1 in, 1 out]
          }
          event "Clear all charts": Value Change {
            (unwired) T30 [] ("History Data")
            w490 = cluster{dbl}[] [] ("History Data")
            w491 = cluster{"Resistance":sgl}[] [] ("History Data")
            w488 = dbl[] [] ("History Data")
            n119 = event-data() -> ()  [unwired: 1 in, 1 out]
            n120 = property on="K-6430" class="WFChart (strict)"("History Data"=w491) -> ()  [unwired: 2 in, 2 out]
            n121 = property on="arduino qcm 1" class="WFChart (strict)"("History Data"=w488) -> ()  [unwired: 2 in, 2 out]
            n122 = property on="Waveform Chart" class="WFChart (strict)"("History Data"=w490) -> ()  [unwired: 2 in, 2 out]
            n123 = property on="arduino qcm 6" class="WFChart (strict)"("History Data"=w488) -> ()  [unwired: 2 in, 2 out]
            n124 = property on="arduino qcm 3" class="WFChart (strict)"("History Data"=w488) -> ()  [unwired: 2 in, 2 out]
            n125 = property on="QCM plot" class="WFChart (strict)"("History Data"=cluster{dbl, "Resistance out":dbl}[] []) -> ()  [unwired: 2 in, 2 out]
            n126 = property on="K-2100 (Ohm)" class="WFChart (strict)"("History Data"=w491) -> ()  [unwired: 2 in, 2 out]
            n127 = property on="arduino qcm 4" class="WFChart (strict)"("History Data"=w488) -> ()  [unwired: 2 in, 2 out]
            n128 = property on="K-2420" class="WFChart (strict)"("History Data"=w491) -> ()  [unwired: 2 in, 2 out]
            n129 = property on="pressure chart" class="WFChart (strict)"("History Data"=w490) -> ()  [unwired: 2 in, 2 out]
            n130 = property on="arduino qcm 2" class="WFChart (strict)"("History Data"=w488) -> ()  [unwired: 2 in, 2 out]
            n131 = property on="arduino qcm 5" class="WFChart (strict)"("History Data"=w488) -> ()  [unwired: 2 in, 2 out]
          }
          event "Sequence cluster.Clear sequence": Value Change {
            n132 = event-data() -> ()  [unwired: 1 in, 1 out]
            n133 = property on="User-defined\nsequence" class="Tbl (strict)"("Value"=string[][] []) -> ()  [unwired: 2 in, 2 out]
          }
          event "Sequence cluster.Save sequence": Value Change {
            n134 = event-data() -> ()  [unwired: 1 in, 1 out]
            n135 = call-poly <vilib>:"Write To Spreadsheet File.vi"("2D data"=w493) -> ()  [unwired: 7 in, 1 out]
          }
          event "Sequence cluster.Import sequence file": Value Change {
            n136 = event-data() -> ()  [unwired: 1 in, 1 out]
            n137 = call-poly <vilib>:"Read From Spreadsheet File.vi"() -> ("all rows"=w494:string[][])  [unwired: 7 in, 4 out]
            n138 = property on="User-defined\nsequence" class="Tbl (strict)"("Value"=w494) -> ()  [unwired: 2 in, 2 out]
          }
        }
        n139 = Unbundle(w327) -> ("press/RH/gas/vapor"=w326:T31, "Cluster"=w325:T32)
        n140 = Fract/Exp String To Number(string=w308) -> (number=w303:T33)  [unwired: 3 in, 1 out]
        n141 = Unbundle(w325) -> ("Valve position (%)"=w323:dbl, "read pressure"=w317:dbl, "read vapor flow"=w322:dbl, "read gas flow"=w321:dbl)
        n142 = Unbundle("Data logging settings") -> ("Save during sequence only"=w400:bool, "Save now"=w402:bool, "sec between data points"=w389:dbl, "Save sample names"=w344:T34, "Experiment Notes"=w343:string)  [unwired: 1 out]
        n143 = property on="Valve position (%)" class="DigNum (strict)"("Value"=w323) -> ()  [unwired: 2 in, 2 out]
        n144 = case shown="True" w305 {
          tunnel: w303 -> [_ w473]
          frame False {
          }
          frame True {
            n145 = Unbundle(w473) -> ("mean"=w472:dbl, "mean"=w471:dbl, "mean"=w470:dbl, "mean"=w469:dbl, "mean"=w468:dbl, "mean"=w466:dbl)
            n146 = Bundle("mean"=w472, "mean"=w472, "mean"=w471, "mean"=w471, "mean"=w470, "mean"=w470, "mean"=w469, "mean"=w469, "mean"=w468, "mean"=w468, "mean"=w466, "mean"=w466) -> (→"ArduinoQCM\ncluster":T35)  [unwired: 1 in]
          }
        }
        n147 = Subtract(x=w387, y=w368) -> (x-y=w386:dbl)
        n148 = property on="read pressure" class="DigNum (strict)"("Value"=w317) -> ()  [unwired: 2 in, 2 out]
        n149 = And(x=w324, y=w400) -> (x .and. y?=w399:bool)
        n150 = case shown="True" w283 {
          tunnel: w294 -> [w446 w449]
          tunnel: w293 -> [w445 w450]
          tunnel: [w446 w448] -> w291
          tunnel: [w445 w447] -> w292
          frame False {
          }
          frame True {
            n151 = Concatenate Strings("#000TMPOFF" ("write buffer 2"), "\r", "\n") -> (w451:string)
            n152 = VISA Write(VISA resource name=w449, write buffer=w451, error in (no error)=w450) -> (VISA resource name out=w448:refnum<visa-resource-name>, error out=w447:errorcluster)  [unwired: 1 out]
          }
        }
        n153 = Bundle("read pressure"=w317) -> (w316:cluster{"read pressure":dbl})  [unwired: 1 in]
        n154 = Divide(x=w386, y=60.0) -> (x/y=w360:dbl)
        "Elapsed time (min)" <- w360
        n155 = call "data_headers_subVI.vi"("Experiment Notes"=w343, "Sample names"=w344) -> ("data headers"=w413:string[])  [unwired: 9 in]
        n156 = property on="read vapor flow" class="DigNum (strict)"("Value"=w322) -> ()  [unwired: 2 in, 2 out]
        n157 = Multiply(x=w389, y=u32 1000 ("x")) -> (x*y=w422:dbl)
        n158 = Or(x=w399, y=w402) -> (x .or. y?=w396:bool)
        "saving data?" <- w396
        n159 = Wait (ms)(milliseconds to wait=w422) -> ()  [unwired: 1 out]
        n160 = property on="read gas flow" class="DigNum (strict)"("Value"=w321) -> ()  [unwired: 2 in, 2 out]
        n161 = property on="pressure chart" class="WFChart (strict)"("Value"=w316) -> ()  [unwired: 2 in, 2 out]
        n162 = Get Date/Time In Seconds() -> (seconds since 1Jan1904=w444:timestamp)
        n163 = Number To Engineering String ("elapsed time (min)")(4:w360) -> (0:w365:string)  [unwired: 3 in]
        n164 = Unbundle(w339) -> ("current  step # in"=w314:i32, "sequence end time in"=w338:timestamp, "Boolean"=w337:bool)
        n165 = Format Date/Time String(time format string (%c)="%Y-%m-%d %H:%M:%S%2u", seconds (now)=w444) -> (date/time string=w419:string)  [unwired: 1 in]
        n166 = Unbundle(w373) -> ("String data out"=w364:string, w363:string, w362:string, w361:string)
        n167 = Unbundle(w418) -> ("String"=w366:string, "String"=w421:string, "String"=w420:string)
        n168 = Unbundle(w357) -> ("String"=w356:string, "String"=w355:string)
        n169 = Unbundle(w326) -> ("pressure"=w412:string, "RH"=w411:string, "gas flow"=w410:string, "vapor flow"=w409:string)
        n170 = Unbundle ("arduino 1-6")(w308) -> ("mean"=w312:string, "mean"=w417:string, "mean"=w416:string, "mean"=w415:string, "mean"=w414:string, "mean"=w310:string)
        n171 = Increment(x=w314) -> (x+1=w313:i32)
        n172 = Build Array(w419, w365, w364, w363, w362, w361, w366, w421, w420, w356, w355, w412, w411, w410, w409, w311, w312, w417, w416, w415, w414, w310) -> (w427:string[])
        n173 = property on="Current\nstep" class="DigNum (strict)"("Value"=w313) -> ()  [unwired: 2 in, 2 out]
        "State date/time" <- w359
      }
      n174 = Unbundle(w88) -> (w87:bool, "VISA resource name out"=w86:refnum<visa-resource-name>, "error out"=w85:errorcluster)
      n175 = Unbundle(w84) -> ("Boolean"=w83:bool, "VISA out"=w82:refnum<visa-resource-name>, "error out"=w81:errorcluster)
      n176 = call-poly <vilib>:"Write To Spreadsheet File.vi"("1D data"=w52, "file path (dialog if empty)"=w69) -> ("new file path (Not A Path if cancelled)"=w73:path)  [unwired: 6 in]
      n177 = Unbundle(w62) -> (w67:bool, "VISA resource name out"=w66:refnum<visa-resource-name>, "error out"=w65:errorcluster)
      n178 = Unbundle(w33) -> ("Boolean"=w32:bool, "task out"=w14:refnum<k21>, "error out"=w13:errorcluster, "task out"=w12:refnum<k21>, "error out"=w11:errorcluster, "VISA resource name out"=w10:refnum<visa-resource-name>, "error out"=w9:errorcluster)
      n179 = call "arduino_close_subIV.vi"("arduino 1-6 addresses and errors out"=w54, "arduinos on?"=w53) -> ()  [unwired: 10 in]
      n180 = case shown="True" w45 {
        tunnel: w44 -> [_ w108]
        tunnel: w43 -> [w105 w107]
        tunnel: [w105 w106] -> w42
        frame False {
        }
        frame True {
          n181 = call "Close.vi"("VISA resource name"=w108, "error in (no error)"=w107) -> ("error out"=w106:errorcluster)  [unwired: 17 in]
        }
      }
      n182 = flat-sequence {
        tunnel: w19 -> [w104]
        tunnel: [w104] -> w18
        frame #0 {
          n183 = property on="saving data?" class="Bool (strict)"("Value"=FALSE ("saving data?")) -> ()  [unwired: 2 in, 2 out]
        }
      }
      n184 = Unbundle(w79) -> ("Boolean"=w78:bool, "VISA resource name out"=w77:refnum<visa-resource-name>, "error out"=w76:errorcluster)
      n185 = case shown="True" w32 {
        tunnel: [errorcluster {"status"=FALSE, "code"=0, "source"=""} ("error out") w133] -> w37
        tunnel: w14 -> [_ w132]
        tunnel: w13 -> [_ w131]
        tunnel: w12 -> [_ w130]
        tunnel: w11 -> [_ w127]
        tunnel: w10 -> [_ w128]
        tunnel: w9 -> [_ w129]
        tunnel: w5 -> [_ w124]
        tunnel: w4 -> [_ w123]
        frame False {
        }
        frame True {
          n186 = call <vilib>:"DAQmx Stop Task.vi"("task/channels in"=w132, "error in"=w131) -> ("task out"=w139:refnum<k21>, "error out"=w138:errorcluster)  [unwired: 12 in]
          n187 = call <vilib>:"DAQmx Stop Task.vi"("task/channels in"=w130, "error in"=w127) -> ("task out"=w140:refnum<k21>, "error out"=w141:errorcluster)  [unwired: 12 in]
          n188 = VISA Clear(VISA resource name=w128, error in (no error)=w129) -> (VISA resource name out=w137:refnum<visa-resource-name>, error out=w136:errorcluster)
          n189 = VISA Close(VISA resource name=w124, error in (no error)=w123) -> (error out=w125:errorcluster)
          n190 = VISA Close(VISA resource name=w137, error in (no error)=w136) -> (error out=w126:errorcluster)
          n191 = call <vilib>:"DAQmx Clear Task.vi"("task in"=w139, "error in"=w138) -> ("error out"=w135:errorcluster)  [unwired: 13 in]
          n192 = call <vilib>:"DAQmx Clear Task.vi"("task in"=w140, "error in"=w141) -> ("error out"=w134:errorcluster)  [unwired: 13 in]
          n193 = Merge Errors(w135, w134, w126, w125) -> (w133:errorcluster)
        }
      }
      n194 = case shown="True" w87 {
        tunnel: w86 -> [_ w257]
        tunnel: w85 -> [w254 w256]
        tunnel: [w254 w255] -> w89
        frame False {
        }
        frame True {
          n195 = call "Enable Output.vi"("error in (no error)"=w256, "Enable Output (T: Enable)"=FALSE, "VISA resource name"=w257) -> ("error out"=w258:errorcluster, "VISA resource name out"=w260:refnum<visa-resource-name>)  [unwired: 7 in]
          n196 = call "Close.vi"("error in (no error)"=w258, "VISA resource name"=w260) -> ("error out"=w255:errorcluster)  [unwired: 9 in]
        }
      }
      n197 = case shown="True" w67 {
        tunnel: w66 -> [_ w172]
        tunnel: w65 -> [w170 w171]
        tunnel: [w170 w173] -> w61
        frame False {
        }
        frame True {
          n198 = call "Enable Output.vi"("error in (no error)"=w171, "Enable Output (F:Off)"=FALSE ("Output (F:Off)"), "VISA resource name"=w172) -> ("error out"=w174:errorcluster, "VISA resource name out"=w175:refnum<visa-resource-name>)  [unwired: 7 out]
          n199 = call "Close.vi"("error in (no error)"=w174, "VISA resource name"=w175) -> ("error out"=w173:errorcluster)  [unwired: 9 out]
        }
      }
      n200 = case shown="True" w83 {
        tunnel: w81 -> [w240 w243]
        tunnel: [w240 w242] -> w90
        tunnel: w82 -> [_ w241]
        frame False {
        }
        frame True {
          n201 = call "srsQcm200Close.vi"("error in"=w243, "Visa in"=w241) -> ("error out"=w242:errorcluster)  [unwired: 3 in]
        }
      }
      n202 = call-poly <vilib>:"Write To Spreadsheet File.vi"("append to file? (new file:F)"=TRUE, "2D data"=w56, "file path (dialog if empty)"=w73) -> ()  [unwired: 5 in, 1 out]
      n203 = case shown="True" w78 {
        tunnel: w77 -> [_ w210]
        tunnel: w76 -> [w207 w209]
        tunnel: [w207 w208] -> w75
        frame False {
        }
        frame True {
          n204 = VISA Close(VISA resource name=w210, error in (no error)=w209) -> (error out=w208:errorcluster)
        }
      }
      n205 = Merge Errors(w61, w75, w89, w42, w90, w18) -> (w96:errorcluster)
      n206 = call <vilib>:"Simple Error Handler.vi"("error in (no error)"=w37) -> ()  [unwired: 4 in, 5 out]
      n207 = call <vilib>:"Simple Error Handler.vi"("error in (no error)"=w96) -> ()  [unwired: 4 in, 5 out]
    }
  }
